vi "Templates_Set Active Data BG Color.vi"(7 "Highlight Color":T1, 8 "error in":errorcluster, 9 "Active Data":variant, 11 "Ctl Refnum":refnum<vi>) -> (0 "error out":errorcluster, 1 "Active Data":variant, 2 "Label":string)   [LabVIEW 2021, in "FakedArray.lvclass"]
uses:
  <resource>/plugins/NIIconEditor/Class/FakedArray/FakedArray.lvclass
  <vilib>/LabVIEW Icon API/lv_icon/Controls/Graphic.ctl
  <vilib>/LabVIEW Icon API/lv_icon/Controls/IEColor.ctl
panel:
  in  "?":T2
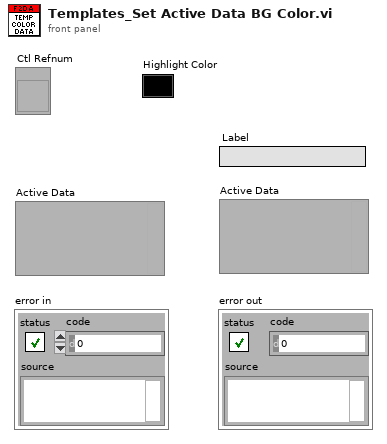
[diagram p1: front panel]
types:
  T1 = typedef "IEColor.ctl" = u32
  T2 = typedef "Graphic.ctl" = cluster{"Rectangle":cluster{"left":i16, "top":i16, "right":i16, "bottom":i16}, "Path":path, "Image":picture, "Filter":string, "FileName":string}
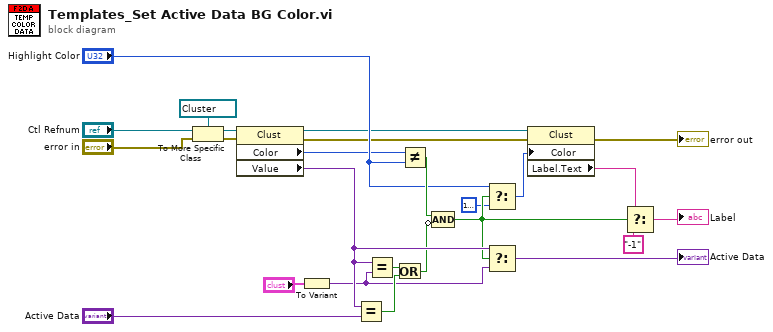
[diagram p0: block diagram]
diagram:
  n1 = To More Specific Class(target class=refnum<vi> refnum ("Clust Refnum"), reference="Ctl Refnum", error in="error in") -> (specific class reference=w9:refnum<vi>, error out=w4:errorcluster)
  n2 = property class="Clust"(reference=w9, error in=w4) -> (reference out=w6:refnum<vi>, error out=w7:errorcluster, "Color"=w5:u32, "Value"=w25:variant)
  n3 = To Variant(anything="?") -> (Variant=w21:variant)
  n4 = Equal?(x=w25, y="Active Data") -> (x = y?=w23:bool)
  n5 = Equal?(x=w25, y=w21) -> (x = y?=w20:bool)
  n6 = Or(x=w20, y=w23) -> (x .or. y?=w24:bool)
  n7 = Not Equal?(x=w5, y="Highlight Color") -> (x != y?=w16:bool)
  n8 = Compound Arithmetic op=AND(w16, invert w24) -> (w17:bool)
  n9 = Select(t="Highlight Color", s=w17, f=T1 16777216 ("t")) -> (s? t:f=w8:T1)
  n10 = Select(t=w25, s=w17, f=w21) -> (s? t:f=→"Active Data":variant)
  n11 = property class="Clust"(reference=w6, error in=w7, "Color"=w8) -> (error out=→"error out":errorcluster, "Label.Text"=w13:string)  [unwired: 1 out]
  n12 = Select(t=w13, s=w17, f="-1") -> (s? t:f=→"Label":string)
